vi "Read Data.vi"(11 "NeedleValve in":refnum<class "NeedleValve.lvclass">) -> (2 "data value":T1={"Engine State"=8, "StateValveModbus"=enum."STOPED", "Alarms"={"OL"=FALSE, "TF"=FALSE, "STL"=FALSE, "OCP"=FALSE, "CPUV"=FALSE, "UVLO"=FALSE, "SPI_ERROR"=FALSE, "Fault"=FALSE, "OL 2"=FALSE, "TF 2"=FALSE, "STL 2"=FALSE, "OCP 2"=FALSE, "CPUV 2"=FALSE, "UVLO 2"=FALSE, "reserved"=TRUE, "InitDone"=TRUE}, "RAW"=124110, "Angele"=0.0, "Step"=0, "Encoder"=0, "Kinematic"={"ACC Steps Per Sec^2"=100, "DEC Steps Per Sec^2"=100, "Min Velosity Step Per Sec"=100, "Max Velosity Step Per Sec"=200, "MicroStep"=16}, "Limits"={"Fault 2 Switch"=FALSE, "Fault 1 Switch"=FALSE, "Center(Home)"=FALSE, "Lower Limit"=FALSE, "Upper Limit"=FALSE}, "EncoderMax"=0, "Counter Max Dont Update"=0, "EncoderMin"=0, "Counter Min Dont Update"=0, "Prepere Counter"=0, "STEP INIT"=0, "offset - Angel"=0.0} {"Engine State" items=["ACCELERATING", "DECELERATINGTOSTOP", "DECELERATING", "STEADY", "INDEX_ACCEL", "NDEX_RUN", "INDEX_DECEL", "INDEX_DWELL", "INACTIVE", "STANDBY", "STANDBYTOINACTIVE"]})   [LabVIEW 2019, in "NeedleValve.lvclass"]
uses:
  NeedleValve.lvclass
  TypeDef/Needle Valve Data.ctl
  modbus engine custom/MB_ENGINE_class/Engine State.ctl
  TypeDef/Needle Valve State.ctl
  modbus engine custom/MB_ENGINE_class/Engine Alarms.ctl
  modbus engine custom/MB_ENGINE_class/Settings.ctl
  modbus engine custom/MB_ENGINE_class/Limits Status.ctl
  NeedleValve.lvclass/NeedleValve.ctl
  modbus engine custom/MB_ENGINE_class/MB_ENGINE.lvclass
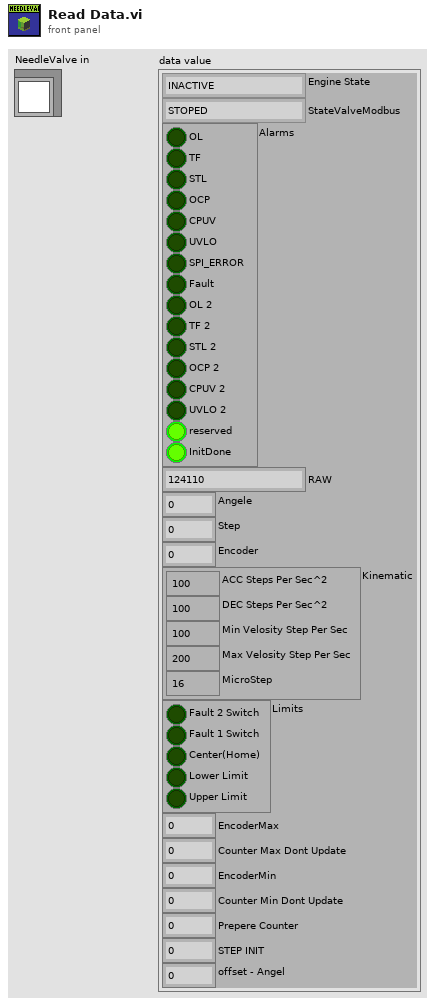
[diagram p1: front panel]
types:
  T1 = typedef "Needle Valve Data.ctl" = cluster{"Engine State":T2, "StateValveModbus":T3, "Alarms":T4, "RAW":i32, "Angele":dbl, "Step":i32, "Encoder":i32, "Kinematic":T5, "Limits":T6, "EncoderMax":i32, "Counter Max Dont Update":i32, "EncoderMin":i32, "Counter Min Dont Update":i32, "Prepere Counter":i32, "STEP INIT":i32, "offset - Angel":dbl}
  T2 = typedef "MB_ENGINE.lvclass/Engine State.ctl" = u16
  T3 = typedef "Needle Valve State.ctl" = enum16{"STOPED", "CLOSED", "OPENED", "OPENING", "CLOSING", "FULL_CLOSE", "PREP_OPEN"}
  T4 = typedef "MB_ENGINE.lvclass/Engine Alarms.ctl" = cluster{"OL":bool, "TF":bool, "STL":bool, "OCP":bool, "CPUV":bool, "UVLO":bool, "SPI_ERROR":bool, "Fault":bool, "OL 2":bool, "TF 2":bool, "STL 2":bool, "OCP 2":bool, "CPUV 2":bool, "UVLO 2":bool, "reserved":bool, "InitDone":bool}
  T5 = typedef "MB_ENGINE.lvclass/Settings.ctl" = cluster{"ACC Steps Per Sec^2":u16, "DEC Steps Per Sec^2":u16, "Min Velosity Step Per Sec":u16, "Max Velosity Step Per Sec":u16, "MicroStep":u16}
  T6 = typedef "MB_ENGINE.lvclass/Limits Status.ctl" = cluster{"Fault 2 Switch":bool, "Fault 1 Switch":bool, "Center(Home)":bool, "Lower Limit":bool, "Upper Limit":bool}
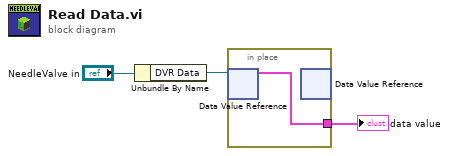
[diagram p0: block diagram]
diagram:
  n1 = Unbundle By Name("NeedleValve in") -> ("DVR Data"=w2:refnum<data-value>)
  n2 = in-place {
    in-place-border: [w4] -> w1
    n3 = in-place-dvr #1(w2) -> (w4:T1)  [unwired: 1 out]
    n4 = in-place-dvr #1() -> ()  [unwired: 1 in, 2 out]
  }
  "data value" <- w1
